vi "generateDataPath.vi"() -> (0 "连接的字符串":string)   [LabVIEW 2018]
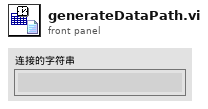
[diagram p1: front panel]
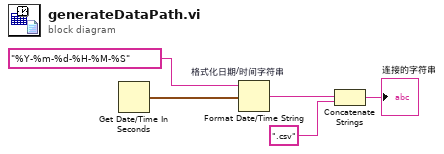
[diagram p0: block diagram]
diagram:
  n1 = Get Date/Time In Seconds() -> (seconds since 1Jan1904=w3:timestamp)
  n2 = Format Date/Time String "格式化日期/时间字符串"(time format string (%c)="%Y-%m-%d-%H-%M-%S" ("时间格式字符串(%c)"), seconds (now)=w3) -> (date/time string=w1:string)  [unwired: 1 in]
  n3 = Concatenate Strings(w1, ".csv" ("字符串")) -> (→"连接的字符串":string)
